vi "dm06_lk_ratio_cal.vi"(8 "Signal power input":dbl[](array[numeric]), 11 "Wavelength_input":dbl[](array[numeric])) -> (3 "Locking ratio [%]":dbl)   [LabVIEW 2020]
uses:
  <vilib>/Analysis/NI_AALBase.lvlib
panel:
  out "Signal with noise reduction":dbl[](array[numeric])
  out "standard deviation":dbl format="%0.2f"
  out "mean":dbl format="%0.2f"
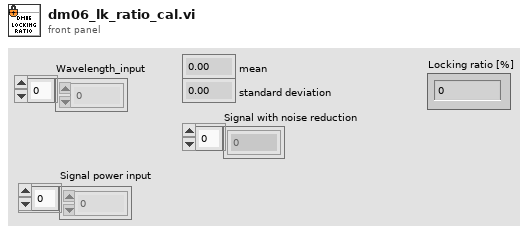
[diagram p1: front panel]
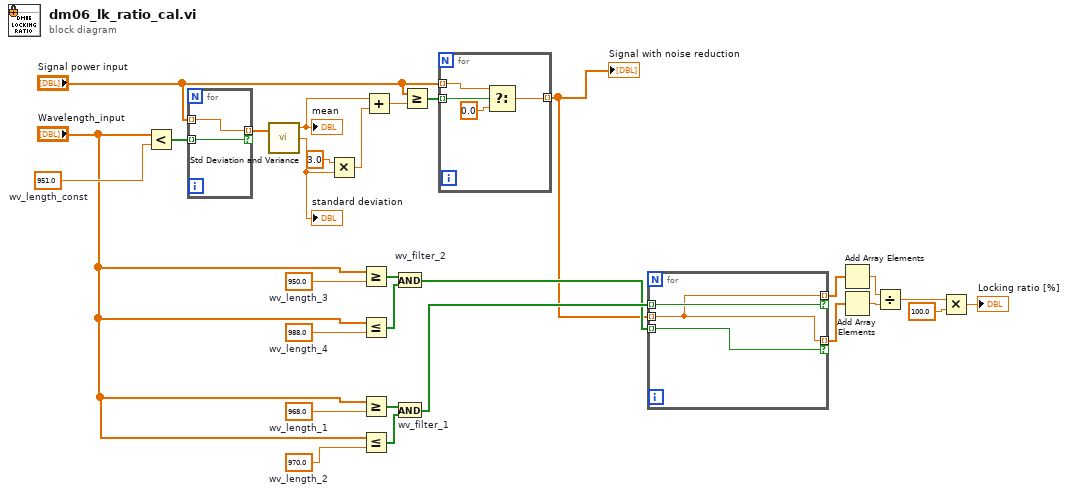
[diagram p0: block diagram]
diagram:
  w15 = 988.0  # wv_length_4
  w16 = 950.0  # wv_length_3
  w1 = 970.0  # wv_length_2
  w19 = 968.0  # wv_length_1
  w29 = 951.0  # wv_length_const
  n1 = Less?(x="Wavelength_input", y=w29) -> (x < y?=w28:bool[])
  n2 = for {
    tunnel: "Signal power input" -> [w31] mode=indexing
    tunnel: w28 -> [w30] mode=indexing
    tunnel: [w31] -> w27 mode=indexing if=w30
  }
  n3 = call <vilib>:"Std Deviation and Variance.vi"("X"=w27) -> ("mean"=w26:dbl, "standard deviation"=w25:dbl)  [unwired: 1 in, 1 out]
  "mean" <- w26
  "standard deviation" <- w25
  n4 = Multiply(x=3.0, y=w25) -> (x*y=w23:dbl)
  n5 = Greater Or Equal?(x="Wavelength_input", y=w16) -> (x >= y?=w14:bool[])
  n6 = Less Or Equal?(x="Wavelength_input", y=w15) -> (x <= y?=w13:bool[])
  n7 = Greater Or Equal?(x="Wavelength_input", y=w19) -> (x >= y?=w18:bool[])
  n8 = Less Or Equal?(x="Wavelength_input", y=w1) -> (x <= y?=w17:bool[])
  n9 = Add(x=w26, y=w23) -> (x+y=w22:dbl)
  n10 = And "wv_filter_2"(x=w14, y=w13) -> (x .and. y?=w11:bool[])
  n11 = And "wv_filter_1"(x=w18, y=w17) -> (x .and. y?=w12:bool[])
  n12 = Greater Or Equal?(x="Signal power input", y=w22) -> (x >= y?=w21:bool[])
  n13 = for {
    tunnel: w21 -> [w35] mode=indexing
    tunnel: "Signal power input" -> [w34] mode=indexing
    tunnel: [w32] -> w5 mode=indexing
    n14 = Select(t=w34, s=w35, f=0.0) -> (s? t:f=w32:dbl)
  }
  "Signal with noise reduction" <- w5
  n15 = for {
    tunnel: w5 -> [w36] mode=indexing
    tunnel: w12 -> [w38] mode=indexing
    tunnel: w11 -> [w37] mode=indexing
    tunnel: [w36] -> w4 mode=indexing if=w38
    tunnel: [w36] -> w3 mode=indexing if=w37
  }
  n16 = Add Array Elements(numeric array=w4) -> (sum=w10:dbl)
  n17 = Add Array Elements(numeric array=w3) -> (sum=w9:dbl)
  n18 = Divide(x=w10, y=w9) -> (x/y=w8:dbl)
  n19 = Multiply(x=w8, y=100.0) -> (x*y=→"Locking ratio [%]":dbl)
